vi "cHECK_Barcode.vi"(10 "Scanned Barcode":string, 11 "Required Barcode":string) -> (3 "Enable?":bool)   [LabVIEW 2020]
uses:
  <userlib>/_OpenG.lib/comparison/comparison.llb/String Changed__ogtk.vi
  <userlib>/_OpenG.lib/comparison/comparison.llb/Boolean Changed__ogtk.vi
  <vilib>/ethernetip/ethernetip.llb/EthernetIP Tag Write BOOL.vi
  <vilib>/ethernetip/ethernetip.llb/EthernetIP Tag Write STRING.vi
  <vilib>/ethernetip/ethernetip.lvlib
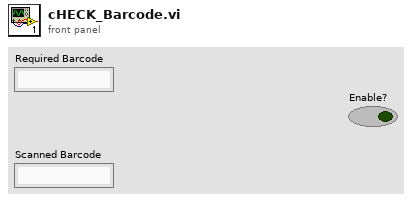
[diagram p1: front panel]
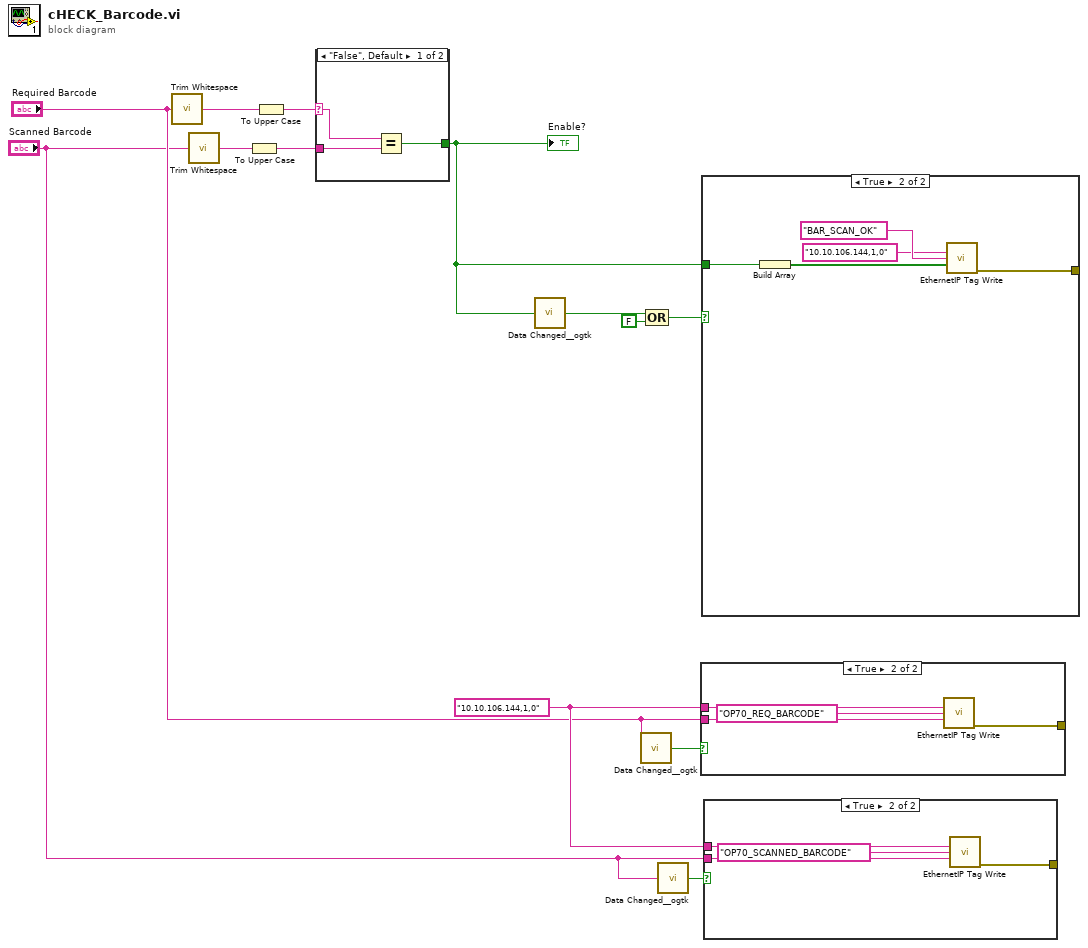
[diagram p0: block diagram]
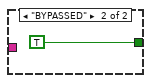
[diagram p5: hidden frame]
diagram:
  w5 = "10.10.106.144,1,0" ("Network Path")
  n1 = call <vilib>:"Trim Whitespace.vi"("string"="Required Barcode") -> ("trimmed string"=w11:string)  [unwired: 1 in]
  n2 = call <vilib>:"Trim Whitespace.vi"("string"="Scanned Barcode") -> ("trimmed string"=w10:string)  [unwired: 1 in]
  n3 = To Upper Case(1:w10) -> (0:w12:string)
  n4 = To Upper Case(1:w11) -> (0:w13:string)
  n5 = case shown="\"False\", Default" w13 {
    selector: w13 -> [w16 _]
    tunnel: [w14 TRUE ("Enable?")] -> w9
    tunnel: w12 -> [w15 _]
    frame "False", Default {
      n6 = Equal?(x=w16, y=w15) -> (x = y?=w14:bool)
    }
    frame "BYPASSED" {
    }
  }
  "Enable?" <- w9
  n7 = call-poly <userlib>:"Data Changed__ogtk.vi"("Boolean"=w9) -> ("Changed"=w8:bool)
  n8 = call-poly <userlib>:"Data Changed__ogtk.vi"("String"="Required Barcode") -> ("Changed"=w3:bool)
  n9 = Compound Arithmetic op=OR(w8, FALSE ("value")) -> (w7:bool)
  n10 = call-poly <userlib>:"Data Changed__ogtk.vi"("String"="Scanned Barcode") -> ("Changed"=w1:bool)
  n11 = case shown="True" w3 {
    tunnel: w5 -> [_ w20]
    tunnel: "Required Barcode" -> [_ w19]
    tunnel: [_ w18] -> _
    frame False {
    }
    frame True {
      n12 = call-poly <vilib>:"EthernetIP Tag Write.vi"("Network Path"=w20, "Tag Name"="OP70_REQ_BARCODE", "Data"=w19) -> ("error out"=w18:errorcluster)  [unwired: 11 in, 1 out]
    }
  }
  n13 = case shown="True" w7 {
    tunnel: w9 -> [_ w24]
    tunnel: [_ w23] -> _
    frame False {
    }
    frame True {
      n14 = Build Array(w24) -> (w25:bool[])
      n15 = call-poly <vilib>:"EthernetIP Tag Write.vi"("Network Path"="10.10.106.144,1,0", "Tag Name"="BAR_SCAN_OK", "Data"=w25) -> ("error out"=w23:errorcluster)  [unwired: 11 in, 1 out]
    }
  }
  n16 = case shown="True" w1 {
    tunnel: "Scanned Barcode" -> [_ w30]
    tunnel: w5 -> [_ w28]
    tunnel: [_ w27] -> _
    frame False {
    }
    frame True {
      n17 = call-poly <vilib>:"EthernetIP Tag Write.vi"("Network Path"=w28, "Tag Name"="OP70_SCANNED_BARCODE", "Data"=w30) -> ("error out"=w27:errorcluster)  [unwired: 11 in, 1 out]
    }
  }
